vi "make_plot_points_lines.vi"(7 "Points/Lines Properties":T1={"Color"=0, "Antialiasing"=FALSE, "Point Size"=0.0, "Points / Lines"=enum."None", "Point Style"=enum."EmptySquare", "Line Style"=enum."Solid", "Line Width"=0.0}, 9 "Transformation":sgl[][](array[numeric]), 10 "Surface Mesh In":refnum<vi>, 11 "Plot Scene Object In":refnum<vi>) -> (1 "Unscaled PL":refnum<vi>, 2 "Drawable":refnum<vi>, 3 "Plot Scene Object Out":refnum<vi>, 4 "PL Scene Object Out":refnum<vi>)   [LabVIEW 2020, in "3DPC_SurfacePlot.xctl"]
uses:
  <vilib>/Native 3D Graph/xcontrol/3DPC_SurfacePlot.xctl
  <vilib>/Native 3D Graph/typedefs/prop_plot_point_line.ctl
  <vilib>/picture/3D Picture Control/Object/Create Object (name).vi
  <vilib>/picture/3D Picture Control/NI_3D Picture Control.lvlib
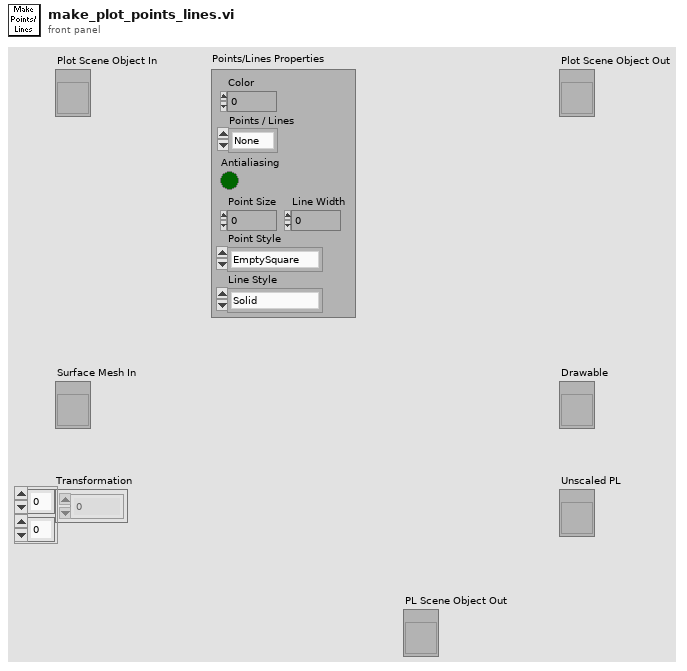
[diagram p1: front panel]
types:
  T1 = typedef "3DPC_SurfacePlot.xctl/prop_plot_point_line.ctl" = cluster{"Color":u32, "Antialiasing":bool, "Point Size":sgl, "Points / Lines":enum16{"None", "Points", "Lines", "Both"}, "Point Style":enum16{"Point", "EmptySquare", "Asterisk", "Diamond", "EmptyCircle", "Circle", "X"}, "Line Style":enum16{"Solid", "Dash", "Dot", "Dash Dot"}, "Line Width":sgl}
  T2 = enum16{"Point", "EmptySquare", "Asterisk", "Diamond", "EmptyCircle", "Circle", "X"}
  T3 = enum16{"Inherit Value", "Points", "Wireframe", "Polygons"}
  T4 = enum16{"Points", "Lines", "Line Strip", "Line Loop", "Triangles", "Triangle Strip", "Triangle Fan", "Quads", "Quad Strip", "Polygon"}
  T5 = enum16{"Overall", "Per Primitive", "Per Vertex", "Binding Off"}
  T6 = typedef "LV3DPointTypeDef.ctl" = cluster{"X":sgl, "Y":sgl, "Z":sgl}
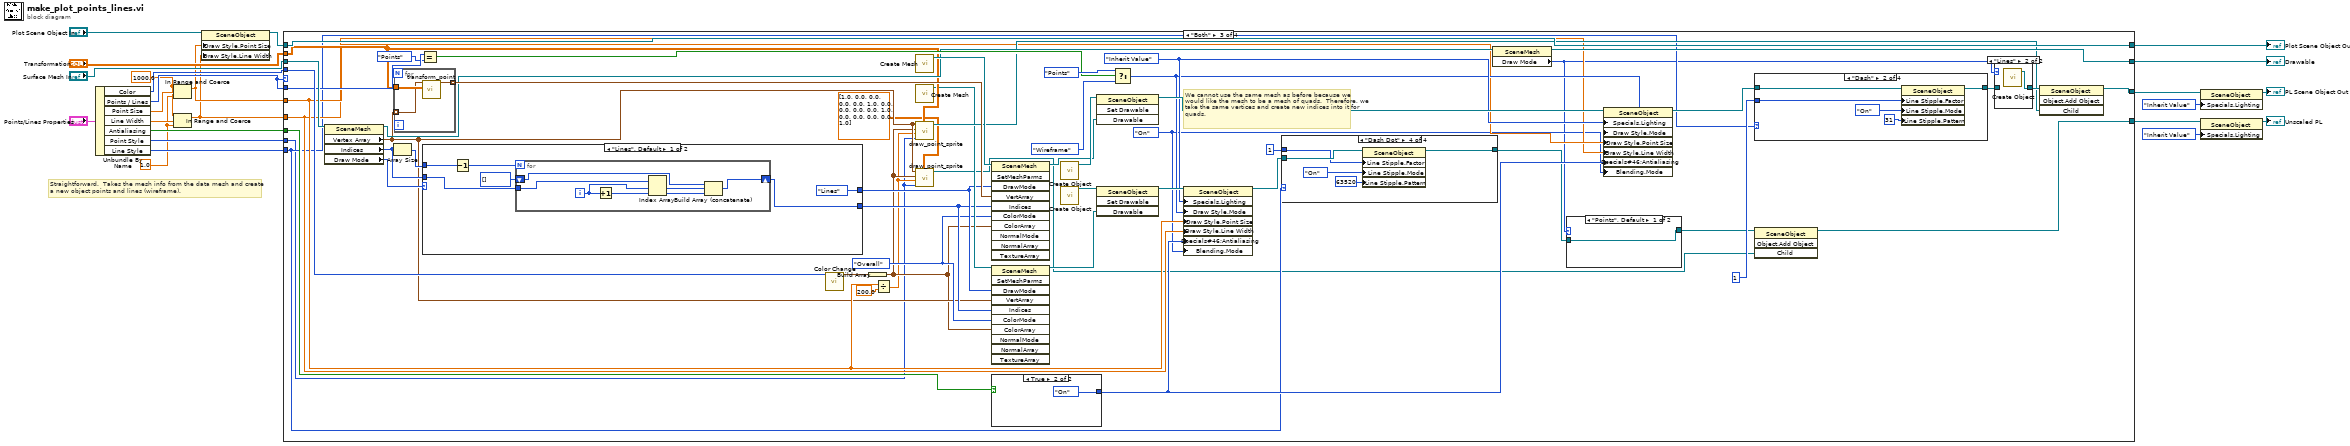
[diagram p0: block diagram]
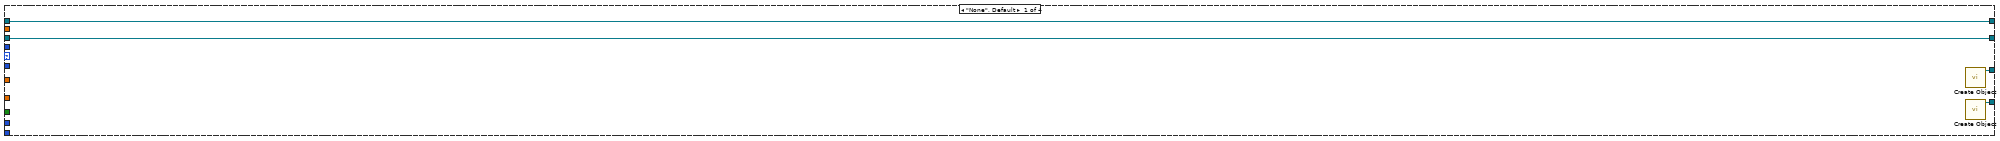
[diagram p2: hidden frame]
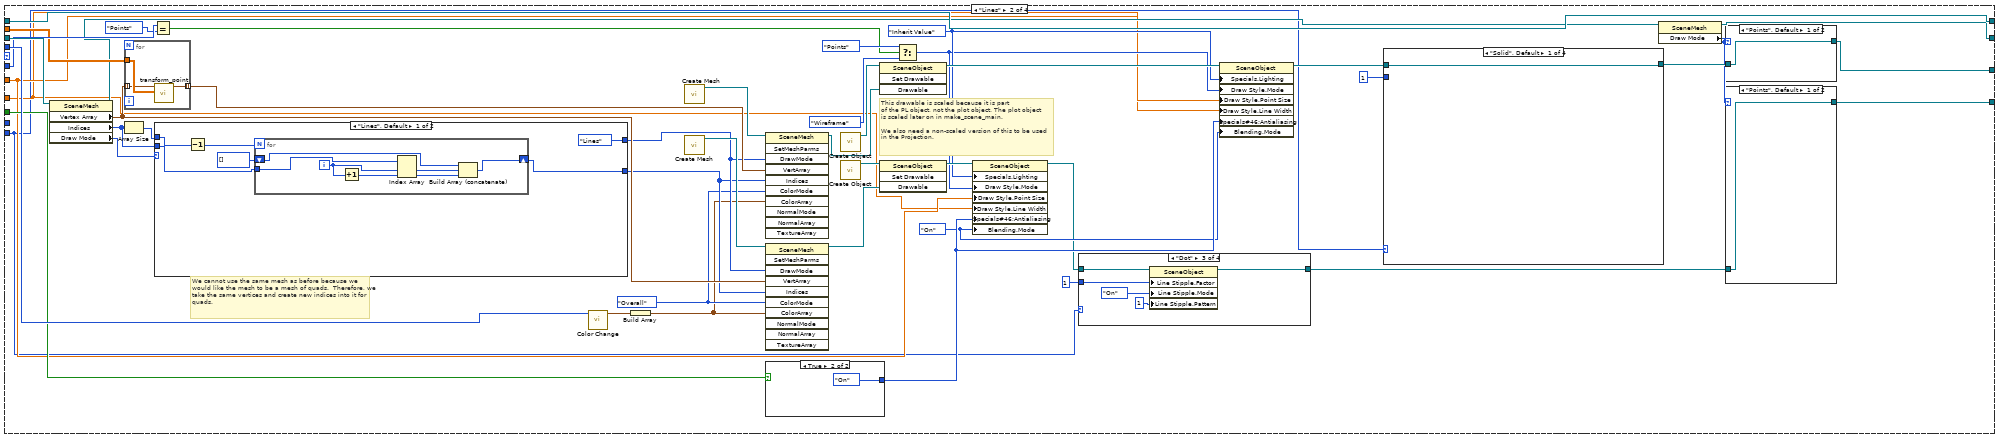
[diagram p3: hidden frame]
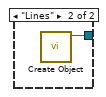
[diagram p4: hidden frame]
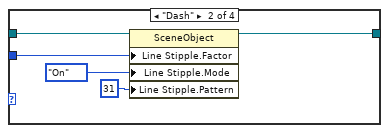
[diagram p6: hidden frame]
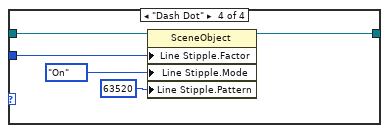
[diagram p7: hidden frame]
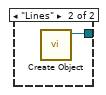
[diagram p8: hidden frame]
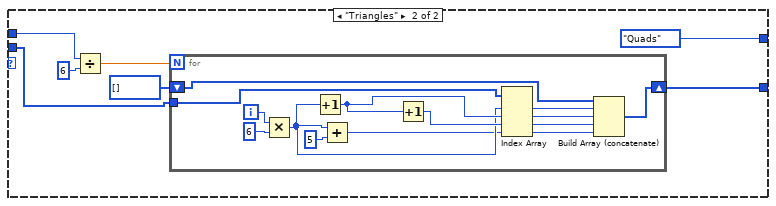
[diagram p9: hidden frame]
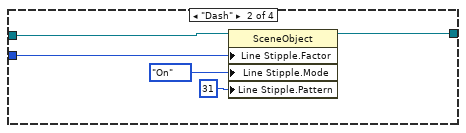
[diagram p10: hidden frame]
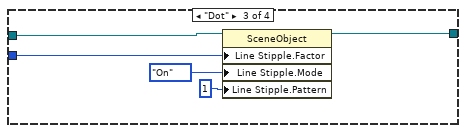
[diagram p11: hidden frame]
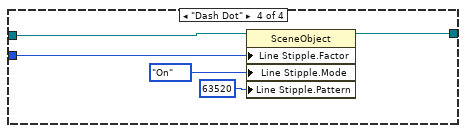
[diagram p12: hidden frame]
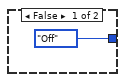
[diagram p13: hidden frame]
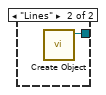
[diagram p14: hidden frame]
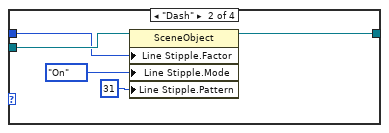
[diagram p16: hidden frame]
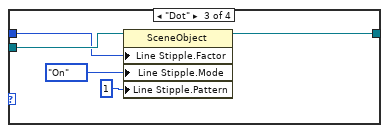
[diagram p17: hidden frame]
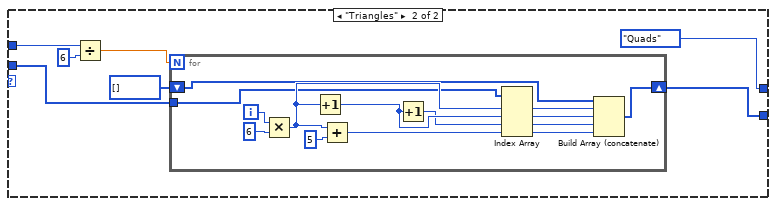
[diagram p19: hidden frame]
diagram:
  w5 = sgl 1000.0 ("upper limit")
  w4 = sgl 1.0 ("lower limit")
  # "Straightforward.  Takes the mesh info from the data mesh and create\na new object points and lines (wireframe)."
  n1 = Unbundle By Name("Points/Lines Properties") -> ("Color"=w22:u32, "Points / Lines"=w18:enum16{"None", "Points", "Lines", "Both"}, "Point Size"=w9:sgl, "Line Width"=w7:sgl, "Antialiasing"=w13:bool, "Point Style"=w16:T2, "Line Style"=w14:enum16{"Solid", "Dash", "Dot", "Dash Dot"})
  n2 = In Range and Coerce(upper limit=w5, x=w9, lower limit=w4) -> (coerced(x)=w8:sgl)  [unwired: 1 out]
  n3 = In Range and Coerce(upper limit=w5, x=w7, lower limit=w4) -> (coerced(x)=w6:sgl)  [unwired: 1 out]
  n4 = property class="SceneObject"(reference="Plot Scene Object In", "Draw Style.Point Size"=w8, "Draw Style.Line Width"=w6) -> (reference out=w17:refnum<vi>)  [unwired: 1 in, 1 out]
  n5 = case shown="\"Both\"" w18 {
    tunnel: "Surface Mesh In" -> [w27 w69 w198 w292]
    tunnel: w22 -> [_ w72 w201 w296]
    tunnel: w18 -> [_ w65 w194 _]
    tunnel: w17 -> [w28 w60 w190 w291]
    tunnel: [w28 w60 w190 w291] -> w21
    tunnel: w8 -> [_ w38 w166 w293]
    tunnel: [w27 w54 w183 w292] -> w19
    tunnel: [w26 w52 w176 w281] -> w12
    tunnel: w13 -> [_ w68 w197 w280]
    tunnel: w16 -> [_ _ w154 w285]
    tunnel: "Transformation" -> [_ w61 w179 w290]
    tunnel: w14 -> [_ w32 w159 _]
    tunnel: w6 -> [_ w37 w165 _]
    tunnel: [w25 w29 w152 w283] -> w3
    frame "None", Default {
      n6 = call-poly <vilib>:"Create Object.vi"() -> ("Scene:New Object"=w26:refnum<vi>)  [unwired: 10 in, 1 out]
      n7 = call-poly <vilib>:"Create Object.vi"() -> ("Scene:New Object"=w25:refnum<vi>)  [unwired: 10 in, 1 out]
    }
    frame "Lines" {
      w35 = enum16{"Inherit Value", "Off", "On"}."On" ("Specials:Antialiasing")
      w46 = T5."Overall" ("Color Binding Mode")
      w40 = enum16{"Inherit Value", "Off", "On"}."Inherit Value" ("Specials:Lighting")
      # "This drawable is scaled because it is part\nof the PL object, not the plot object. The plot object\nis scaled later on in make_scene_main.\n\nWe also need a non-scaled version of this to be used\nin the Projection."
      # "We cannot use the same mesh as before because we would like the mesh to be a mesh of quads.  Therefore, we take the same vertices and create new indices into it for quads."
      n8 = property class="SceneMesh"(reference=w69) -> (reference out=w55:refnum<vi>, "Vertex Array"=w49:T6[], "Indices"=w57:u32[], "Draw Mode"=w56:T4)  [unwired: 1 in, 1 out]
      n9 = for {
        tunnel: w49 -> [w146] mode=indexing
        tunnel: w61 -> [w147]
        tunnel: [w145] -> w62 mode=indexing
        n10 = call <vilib>:"transform_point.vi"("Transformation"=w147, "3D Point"=w146) -> ("output cluster"=w145:T6)  [unwired: 9 out]
      }
      n11 = Array Size(array=w57) -> (size(s)=w58:i32)
      n12 = Equal?(x=w65, y=enum16{"None", "Points", "Lines"}."Points") -> (x = y?=w63:bool)
      n13 = case shown="\"Lines\", Default" w56 {
        tunnel: w58 -> [w97 w112]
        tunnel: w57 -> [w98 w111]
        tunnel: [w96 w110] -> w47
        tunnel: [T4."Lines" ("Draw Mode") T4."Quads" ("Draw Mode")] -> w48
        frame "Lines", Default {
          n14 = Decrement(x=w97) -> (x-1=w100:i32)
          n15 = for {
            N: w100 -> [_]
            tunnel: w98 -> [w104]
            shift-right: [w105] -> w96
            shift-left: u32[] [] ("Indices") -> [w103]
            i -> [w102]
            n16 = Increment(x=w102) -> (x+1=w101:i32)
            n17 = Index Array(array=w104, index #1=w102, index #2=w101) -> (element #1=w107:u32, element #2=w106:u32)
            n18 = Build Array (concatenate)(w103, w107, w106) -> (w105:u32[])
          }
        }
        frame "Triangles" {
          n19 = Divide(x=w112, y=6) -> (x/y=w108:dbl)
          n20 = for {
            N: w108 -> [_]
            tunnel: w111 -> [w116]
            shift-right: [w117] -> w110
            shift-left: u32[] [] ("Indices") -> [w115]
            i -> [w128]
            n21 = Multiply(x=w128, y=6) -> (x*y=w124:i32)
            n22 = Increment(x=w124) -> (x+1=w126:i32)
            n23 = Add(x=w124, y=5) -> (x+y=w122:i32)
            n24 = Increment(x=w126) -> (x+1=w125:i32)
            n25 = Index Array(array=w116, index #1=w124, index #2=w126, index #3=w125, index #4=w122) -> (element #1=w121:u32, element #2=w120:u32, element #3=w119:u32, element #4=w118:u32)
            n26 = Build Array (concatenate)(w115, w121, w120, w119, w118) -> (w117:u32[])
          }
        }
      }
      n27 = call <vilib>:"Color Change.vi"("Color"=w72) -> ("RGBA"=w71:cluster{"R":sgl, "G":sgl, "B":sgl, "A":sgl})  [unwired: 1 in, 9 out]
      n28 = Build Array(w71) -> (w45:cluster{"R":sgl, "G":sgl, "B":sgl, "A":sgl}[])
      n29 = call <vilib>:"Create Mesh.vi"() -> ("New Mesh Refnum"=w70:refnum<vi>)  [unwired: 1 in, 10 out]
      n30 = call <vilib>:"Create Mesh.vi"() -> ("New Mesh Refnum"=w50:refnum<vi>)  [unwired: 1 in, 10 out]
      n31 = invoke class="SceneMesh" method="SetMeshParms"(reference=w70, "DrawMode"=w48, "VertArray"=w62, "Indices"=w47, "ColorMode"=w46, "ColorArray"=w45) -> (reference out=w59:refnum<vi>)  [unwired: 5 in, 10 out]
      n32 = invoke class="SceneMesh" method="SetMeshParms"(reference=w50, "DrawMode"=w48, "VertArray"=w49, "Indices"=w47, "ColorMode"=w46, "ColorArray"=w45) -> (reference out=w43:refnum<vi>)  [unwired: 5 in, 10 out]
      n33 = case shown="True" w68 {
        tunnel: [enum16{"Inherit Value", "Off", "On"}."Off" ("Specials:Antialiasing") enum16{"Inherit Value", "Off", "On"}."On" ("Specials:Antialiasing")] -> w36
        frame False {
        }
        frame True {
        }
      }
      n34 = call-poly <vilib>:"Create Object.vi"() -> ("Scene:New Object"=w74:refnum<vi>)  [unwired: 10 in, 1 out]
      n35 = call-poly <vilib>:"Create Object.vi"() -> ("Scene:New Object"=w44:refnum<vi>)  [unwired: 10 in, 1 out]
      n36 = invoke class="SceneObject" method="Set Drawable"(reference=w74, "Drawable"=w59) -> (reference out=w73:refnum<vi>)  [unwired: 2 in, 3 out]
      n37 = invoke class="SceneObject" method="Set Drawable"(reference=w44, "Drawable"=w43) -> (reference out=w41:refnum<vi>)  [unwired: 2 in, 3 out]
      n38 = Select(t=T3."Points", s=w63, f=T3."Wireframe" ("Draw Style:Mode")) -> (s? t:f=w39:T3)
      n39 = property class="SceneObject"(reference=w41, "Specials.Lighting"=w40, "Draw Style.Mode"=w39, "Draw Style.Point Size"=w38, "Draw Style.Line Width"=w37, "Specials#46;Antialiasing"=w36, "Blending.Mode"=w35) -> (reference out=w34:refnum<vi>)  [unwired: 1 in, 1 out]
      n40 = case shown="\"Dot\"" w32 {
        tunnel: w34 -> [w77 w80 w85 w90]
        tunnel: [w77 w79 w84 w89] -> w30
        tunnel: 1 -> [_ w78 w83 w88]
        frame "Solid", Default {
        }
        frame "Dash" {
          n41 = property class="SceneObject"(reference=w80, "Line Stipple.Factor"=w78, "Line Stipple.Mode"=enum16{"Inherit Value", "Off", "On"}."On" ("Line Stipple:Mode"), "Line Stipple.Pattern"=u16 31 ("Line Stipple:Pattern")) -> (reference out=w79:refnum<vi>)  [unwired: 1 in, 1 out]
        }
        frame "Dot" {
          n42 = property class="SceneObject"(reference=w85, "Line Stipple.Factor"=w83, "Line Stipple.Mode"=enum16{"Inherit Value", "Off", "On"}."On" ("Line Stipple:Mode"), "Line Stipple.Pattern"=u16 1 ("Line Stipple:Pattern")) -> (reference out=w84:refnum<vi>)  [unwired: 1 in, 1 out]
        }
        frame "Dash Dot" {
          n43 = property class="SceneObject"(reference=w90, "Line Stipple.Factor"=w88, "Line Stipple.Mode"=enum16{"Inherit Value", "Off", "On"}."On" ("Line Stipple:Mode"), "Line Stipple.Pattern"=u16 63520 ("Line Stipple:Pattern")) -> (reference out=w89:refnum<vi>)  [unwired: 1 in, 1 out]
        }
      }
      n44 = property class="SceneObject"(reference=w73, "Specials.Lighting"=w40, "Draw Style.Mode"=w39, "Draw Style.Point Size"=w38, "Draw Style.Line Width"=w37, "Specials#46;Antialiasing"=w36, "Blending.Mode"=w35) -> (reference out=w42:refnum<vi>)  [unwired: 1 in, 1 out]
      n45 = case shown="\"Solid\", Default" w32 {
        tunnel: w42 -> [w129 w132 w137 w142]
        tunnel: [w129 w131 w136 w141] -> w53
        tunnel: 1 -> [_ w130 w135 w140]
        frame "Solid", Default {
        }
        frame "Dash" {
          n46 = property class="SceneObject"(reference=w132, "Line Stipple.Factor"=w130, "Line Stipple.Mode"=enum16{"Inherit Value", "Off", "On"}."On" ("Line Stipple:Mode"), "Line Stipple.Pattern"=u16 31 ("Line Stipple:Pattern")) -> (reference out=w131:refnum<vi>)  [unwired: 1 in, 1 out]
        }
        frame "Dot" {
          n47 = property class="SceneObject"(reference=w137, "Line Stipple.Factor"=w135, "Line Stipple.Mode"=enum16{"Inherit Value", "Off", "On"}."On" ("Line Stipple:Mode"), "Line Stipple.Pattern"=u16 1 ("Line Stipple:Pattern")) -> (reference out=w136:refnum<vi>)  [unwired: 1 in, 1 out]
        }
        frame "Dash Dot" {
          n48 = property class="SceneObject"(reference=w142, "Line Stipple.Factor"=w140, "Line Stipple.Mode"=enum16{"Inherit Value", "Off", "On"}."On" ("Line Stipple:Mode"), "Line Stipple.Pattern"=u16 63520 ("Line Stipple:Pattern")) -> (reference out=w141:refnum<vi>)  [unwired: 1 in, 1 out]
        }
      }
      n49 = property class="SceneMesh"(reference=w55) -> (reference out=w54:refnum<vi>, "Draw Mode"=w31:T4)  [unwired: 1 in, 1 out]
      n50 = case shown="\"Points\", Default" w31 {
        tunnel: w53 -> [w93 _]
        tunnel: [w93 w94] -> w52
        frame "Points", Default {
        }
        frame "Lines" {
          n51 = call-poly <vilib>:"Create Object.vi"() -> ("Scene:New Object"=w94:refnum<vi>)  [unwired: 10 in, 1 out]
        }
      }
      n52 = case shown="\"Points\", Default" w31 {
        tunnel: [w75 w76] -> w29
        tunnel: w30 -> [w75 _]
        frame "Points", Default {
        }
        frame "Lines" {
          n53 = call-poly <vilib>:"Create Object.vi"() -> ("Scene:New Object"=w76:refnum<vi>)  [unwired: 10 in, 1 out]
        }
      }
    }
    frame "Both" {
      w163 = enum16{"Inherit Value", "Off", "On"}."On" ("Specials:Antialiasing")
      w169 = T5."Overall" ("Color Binding Mode")
      w168 = enum16{"Inherit Value", "Off", "On"}."Inherit Value" ("Specials:Lighting")
      # "We cannot use the same mesh as before because we would like the mesh to be a mesh of quads.  Therefore, we take the same vertices and create new indices into it for quads."
      n54 = property class="SceneMesh"(reference=w198) -> (reference out=w184:refnum<vi>, "Vertex Array"=w157:T6[], "Indices"=w186:u32[], "Draw Mode"=w185:T4)  [unwired: 1 in, 1 out]
      n55 = for {
        tunnel: w157 -> [w275] mode=indexing
        tunnel: w179 -> [w276]
        tunnel: [w274] -> w191 mode=indexing
        n56 = call <vilib>:"transform_point.vi"("Transformation"=w276, "3D Point"=w275) -> ("output cluster"=w274:T6)  [unwired: 9 out]
      }
      n57 = Array Size(array=w186) -> (size(s)=w187:i32)
      n58 = Equal?(x=w194, y=enum16{"None", "Points", "Lines"}."Points") -> (x = y?=w192:bool)
      n59 = case shown="\"Lines\", Default" w185 {
        tunnel: w187 -> [w226 w241]
        tunnel: w186 -> [w227 w240]
        tunnel: [w225 w239] -> w170
        tunnel: [T4."Lines" ("Draw Mode") T4."Quads" ("Draw Mode")] -> w171
        frame "Lines", Default {
          n60 = Decrement(x=w226) -> (x-1=w229:i32)
          n61 = for {
            N: w229 -> [_]
            tunnel: w227 -> [w233]
            shift-right: [w234] -> w225
            shift-left: u32[] [] ("Indices") -> [w232]
            i -> [w231]
            n62 = Increment(x=w231) -> (x+1=w230:i32)
            n63 = Index Array(array=w233, index #1=w231, index #2=w230) -> (element #1=w236:u32, element #2=w235:u32)
            n64 = Build Array (concatenate)(w232, w236, w235) -> (w234:u32[])
          }
        }
        frame "Triangles" {
          n65 = Divide(x=w241, y=6) -> (x/y=w237:dbl)
          n66 = for {
            N: w237 -> [_]
            tunnel: w240 -> [w245]
            shift-right: [w246] -> w239
            shift-left: u32[] [] ("Indices") -> [w244]
            i -> [w257]
            n67 = Multiply(x=w257, y=6) -> (x*y=w253:i32)
            n68 = Increment(x=w253) -> (x+1=w255:i32)
            n69 = Add(x=w253, y=5) -> (x+y=w251:i32)
            n70 = Increment(x=w255) -> (x+1=w254:i32)
            n71 = Index Array(array=w245, index #1=w253, index #2=w255, index #3=w254, index #4=w251) -> (element #1=w250:u32, element #2=w249:u32, element #3=w248:u32, element #4=w247:u32)
            n72 = Build Array (concatenate)(w244, w250, w249, w248, w247) -> (w246:u32[])
          }
        }
      }
      n73 = call <vilib>:"Color Change.vi"("Color"=w201) -> ("RGBA"=w200:cluster{"R":sgl, "G":sgl, "B":sgl, "A":sgl})  [unwired: 1 in, 9 out]
      n74 = Build Array(w200) -> (w156:cluster{"R":sgl, "G":sgl, "B":sgl, "A":sgl}[])
      n75 = Divide(x=w166, y=sgl 200.0) -> (x/y=w155:sgl)
      n76 = call <vilib>:"Create Mesh.vi"() -> ("New Mesh Refnum"=w199:refnum<vi>)  [unwired: 1 in, 10 out]
      n77 = call <vilib>:"Create Mesh.vi"() -> ("New Mesh Refnum"=w174:refnum<vi>)  [unwired: 1 in, 10 out]
      n78 = call <vilib>:"draw_point_sprite.vi"("Transformation"=w179, "Enum"=w154, "quadsize (4)"=w155, "Color Array"=w156, "Vertex Array"=w157) -> ("Scene:New Object"=w177:refnum<vi>)  [unwired: 6 out]
      n79 = call <vilib>:"draw_point_sprite.vi"("Transformation"=sgl[][] [[1.0, 0.0, 0.0, 0.0], [0.0, 1.0, 0.0, 0.0], [0.0, 0.0, 1.0, 0.0], [0.0, 0.0, 0.0, 1.0]], "Enum"=w154, "quadsize (4)"=w155, "Color Array"=w156, "Vertex Array"=w157) -> ("Scene:New Object"=w151:refnum<vi>)  [unwired: 6 out]
      n80 = invoke class="SceneMesh" method="SetMeshParms"(reference=w199, "DrawMode"=w171, "VertArray"=w191, "Indices"=w170, "ColorMode"=w169, "ColorArray"=w156) -> (reference out=w189:refnum<vi>)  [unwired: 5 in, 10 out]
      n81 = invoke class="SceneMesh" method="SetMeshParms"(reference=w174, "DrawMode"=w171, "VertArray"=w157, "Indices"=w170, "ColorMode"=w169, "ColorArray"=w156) -> (reference out=w173:refnum<vi>)  [unwired: 5 in, 10 out]
      n82 = case shown="True" w197 {
        tunnel: [enum16{"Inherit Value", "Off", "On"}."Off" ("Specials:Antialiasing") enum16{"Inherit Value", "Off", "On"}."On" ("Specials:Antialiasing")] -> w164
        frame False {
        }
        frame True {
        }
      }
      n83 = call-poly <vilib>:"Create Object.vi"() -> ("Scene:New Object"=w203:refnum<vi>)  [unwired: 10 in, 1 out]
      n84 = call-poly <vilib>:"Create Object.vi"() -> ("Scene:New Object"=w175:refnum<vi>)  [unwired: 10 in, 1 out]
      n85 = invoke class="SceneObject" method="Set Drawable"(reference=w203, "Drawable"=w189) -> (reference out=w202:refnum<vi>)  [unwired: 2 in, 3 out]
      n86 = invoke class="SceneObject" method="Set Drawable"(reference=w175, "Drawable"=w173) -> (reference out=w172:refnum<vi>)  [unwired: 2 in, 3 out]
      n87 = Select(t=T3."Points", s=w192, f=T3."Wireframe" ("Draw Style:Mode")) -> (s? t:f=w167:T3)
      n88 = property class="SceneObject"(reference=w172, "Specials.Lighting"=w168, "Draw Style.Mode"=w167, "Draw Style.Point Size"=w166, "Draw Style.Line Width"=w165, "Specials#46;Antialiasing"=w164, "Blending.Mode"=w163) -> (reference out=w162:refnum<vi>)  [unwired: 1 in, 1 out]
      n89 = case shown="\"Dash Dot\"" w159 {
        tunnel: w162 -> [w206 w209 w214 w219]
        tunnel: [w206 w208 w213 w218] -> w160
        tunnel: 1 -> [_ w207 w212 w217]
        frame "Solid", Default {
        }
        frame "Dash" {
          n90 = property class="SceneObject"(reference=w209, "Line Stipple.Factor"=w207, "Line Stipple.Mode"=enum16{"Inherit Value", "Off", "On"}."On" ("Line Stipple:Mode"), "Line Stipple.Pattern"=u16 31 ("Line Stipple:Pattern")) -> (reference out=w208:refnum<vi>)  [unwired: 1 in, 1 out]
        }
        frame "Dot" {
          n91 = property class="SceneObject"(reference=w214, "Line Stipple.Factor"=w212, "Line Stipple.Mode"=enum16{"Inherit Value", "Off", "On"}."On" ("Line Stipple:Mode"), "Line Stipple.Pattern"=u16 1 ("Line Stipple:Pattern")) -> (reference out=w213:refnum<vi>)  [unwired: 1 in, 1 out]
        }
        frame "Dash Dot" {
          n92 = property class="SceneObject"(reference=w219, "Line Stipple.Factor"=w217, "Line Stipple.Mode"=enum16{"Inherit Value", "Off", "On"}."On" ("Line Stipple:Mode"), "Line Stipple.Pattern"=u16 63520 ("Line Stipple:Pattern")) -> (reference out=w218:refnum<vi>)  [unwired: 1 in, 1 out]
        }
      }
      n93 = property class="SceneMesh"(reference=w184) -> (reference out=w183:refnum<vi>, "Draw Mode"=w158:T4)  [unwired: 1 in, 1 out]
      n94 = case shown="\"Points\", Default" w158 {
        tunnel: [w204 w205] -> w150
        tunnel: w160 -> [w204 _]
        frame "Points", Default {
        }
        frame "Lines" {
          n95 = call-poly <vilib>:"Create Object.vi"() -> ("Scene:New Object"=w205:refnum<vi>)  [unwired: 10 in, 1 out]
        }
      }
      n96 = property class="SceneObject"(reference=w202, "Specials.Lighting"=w168, "Draw Style.Mode"=w167, "Draw Style.Point Size"=w166, "Draw Style.Line Width"=w165, "Specials#46;Antialiasing"=w164, "Blending.Mode"=w163) -> (reference out=w188:refnum<vi>)  [unwired: 1 in, 1 out]
      n97 = case shown="\"Dash\"" w159 {
        tunnel: w188 -> [w258 w261 w266 w271]
        tunnel: [w258 w260 w265 w270] -> w182
        tunnel: 1 -> [_ w259 w264 w269]
        frame "Solid", Default {
        }
        frame "Dash" {
          n98 = property class="SceneObject"(reference=w261, "Line Stipple.Factor"=w259, "Line Stipple.Mode"=enum16{"Inherit Value", "Off", "On"}."On" ("Line Stipple:Mode"), "Line Stipple.Pattern"=u16 31 ("Line Stipple:Pattern")) -> (reference out=w260:refnum<vi>)  [unwired: 1 in, 1 out]
        }
        frame "Dot" {
          n99 = property class="SceneObject"(reference=w266, "Line Stipple.Factor"=w264, "Line Stipple.Mode"=enum16{"Inherit Value", "Off", "On"}."On" ("Line Stipple:Mode"), "Line Stipple.Pattern"=u16 1 ("Line Stipple:Pattern")) -> (reference out=w265:refnum<vi>)  [unwired: 1 in, 1 out]
        }
        frame "Dash Dot" {
          n100 = property class="SceneObject"(reference=w271, "Line Stipple.Factor"=w269, "Line Stipple.Mode"=enum16{"Inherit Value", "Off", "On"}."On" ("Line Stipple:Mode"), "Line Stipple.Pattern"=u16 63520 ("Line Stipple:Pattern")) -> (reference out=w270:refnum<vi>)  [unwired: 1 in, 1 out]
        }
      }
      n101 = invoke class="SceneObject" method="Object.Add Object"(reference=w150, "Child"=w151) -> (reference out=w152:refnum<vi>)  [unwired: 2 in, 3 out]
      n102 = case shown="\"Lines\"" w158 {
        tunnel: w182 -> [w222 _]
        tunnel: [w222 w223] -> w178
        frame "Points", Default {
        }
        frame "Lines" {
          n103 = call-poly <vilib>:"Create Object.vi"() -> ("Scene:New Object"=w223:refnum<vi>)  [unwired: 10 in, 1 out]
        }
      }
      n104 = invoke class="SceneObject" method="Object.Add Object"(reference=w178, "Child"=w177) -> (reference out=w176:refnum<vi>)  [unwired: 2 in, 3 out]
    }
    frame "Points" {
      # "We cannot use the same mesh as before because we would like the mesh to be a mesh of quads.  Therefore, we take the same vertices and create new indices into it for quads."
      n105 = property class="SceneMesh"(reference=w292) -> ("Vertex Array"=w288:T6[])  [unwired: 1 in, 2 out]
      n106 = case shown="True" w280 {
        tunnel: [enum16{"Inherit Value", "Off", "On"}."Off" ("Specials:Antialiasing") enum16{"Inherit Value", "Off", "On"}."On" ("Specials:Antialiasing")] -> w279
        frame False {
        }
        frame True {
        }
      }
      n107 = call <vilib>:"Color Change.vi"("Color"=w296) -> ("RGBA"=w295:cluster{"R":sgl, "G":sgl, "B":sgl, "A":sgl})  [unwired: 1 in, 9 out]
      n108 = Build Array(w295) -> (w287:cluster{"R":sgl, "G":sgl, "B":sgl, "A":sgl}[])
      n109 = Divide(x=w293, y=sgl 200.0) -> (x/y=w286:sgl)
      n110 = call <vilib>:"draw_point_sprite.vi"("Transformation"=w290, "Enum"=w285, "quadsize (4)"=w286, "Color Array"=w287, "Vertex Array"=w288) -> ("Scene:New Object"=w282:refnum<vi>)  [unwired: 6 out]
      n111 = call <vilib>:"draw_point_sprite.vi"("Transformation"=sgl[][] [[1.0, 0.0, 0.0, 0.0], [0.0, 1.0, 0.0, 0.0], [0.0, 0.0, 1.0, 0.0], [0.0, 0.0, 0.0, 1.0]], "Enum"=w285, "quadsize (4)"=w286, "Color Array"=w287, "Vertex Array"=w288) -> ("Scene:New Object"=w284:refnum<vi>)  [unwired: 6 out]
      n112 = property class="SceneObject"(reference=w282, "Specials#46;Antialiasing"=w279) -> (reference out=w281:refnum<vi>)  [unwired: 1 in, 1 out]
      n113 = property class="SceneObject"(reference=w284, "Specials#46;Antialiasing"=w279) -> (reference out=w283:refnum<vi>)  [unwired: 1 in, 1 out]
    }
  }
  "Plot Scene Object Out" <- w21
  "Drawable" <- w19
  n114 = property class="SceneObject"(reference=w12, "Specials.Lighting"=enum16{"Inherit Value", "Off", "On"}."Inherit Value" ("Specials:Lighting")) -> (reference out=→"PL Scene Object Out":refnum<vi>)  [unwired: 1 in, 1 out]
  n115 = property class="SceneObject"(reference=w3, "Specials.Lighting"=enum16{"Inherit Value", "Off", "On"}."Inherit Value" ("Specials:Lighting")) -> (reference out=→"Unscaled PL":refnum<vi>)  [unwired: 1 in, 1 out]
